vi "ExtCall.vi"(8 "error in (no error)":errorcluster, 9 "Val":variant, 10 "Tag":u16, 11 "Sine in":refnum<class "Rigol DG822 Sine.lvclass">) -> (0 "error out":errorcluster, 1 "Response":variant, 3 "Sine out":refnum<class "Rigol DG822 Sine.lvclass">)   [LabVIEW 2021, in "Rigol DG822 UI.lvlib" / "Rigol DG822 Sine.lvlib" / "Rigol DG822 Sine.lvclass"]
uses:
  Rigol DG822 Sine.lvclass
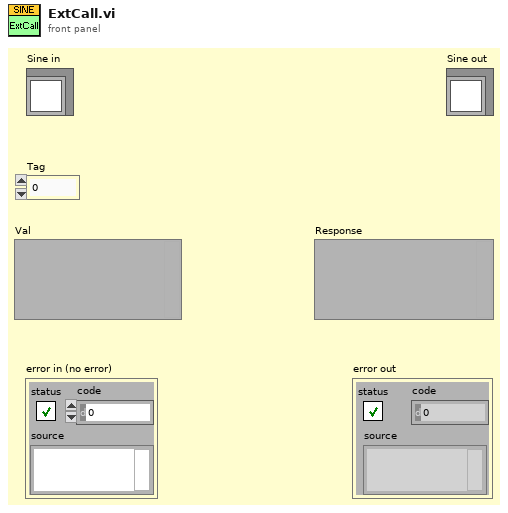
[diagram p1: front panel]
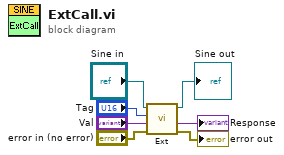
[diagram p0: block diagram]
diagram:
  n1 = call "Ext.vi"("error in (no error)"="error in (no error)", "Val"="Val", "Tag"="Tag", "Sine in"="Sine in") -> ("error out"=→"error out":errorcluster, "Parsed"=→"Response":variant, "Sine out"=→"Sine out":refnum<class "Rigol DG822 Sine.lvclass">)  [unwired: 5 in]
